vi "Agilent 6000 Series Edge Triggered Acquisition.vi"() -> ()   [LabVIEW 2017]
doc: "This example shows how to configure the oscilloscope to perform an edge-triggered waveform acquisition."
uses:
  <instrlib>/Agilent 6000 Series/Public/Configure/Configure Edge Trigger Source.vi
  <instrlib>/Agilent 6000 Series/Public/Data/Read Single Waveform.vi
  <instrlib>/Agilent 6000 Series/Agilent 6000 Series.lvlib
panel:
  in  "Channel (0: Channel 1)":u16(ring) items=["Channel 1", "Channel 2", "Channel 3", "Channel 4"]
  in  "Vertical Coupling (1: DC)":u16(ring)=1 items=["AC", "DC"]
  in  "Probe Attenuation (10.0)":dbl=10.0
  in  "Vertical Range (10.0 V)":dbl=10.0
  in  "Trigger Level (0.5 V)":dbl=0.5
  in  "Timebase (0.0005 s)":dbl=0.0005
  out "Waveform Data":waveform(dbl)(graph)
  in  "VISA resource name":refnum<visa-resource-name>
  # "(c) 2009-2015 National Instruments.  ALL RIGHTS RESERVED."
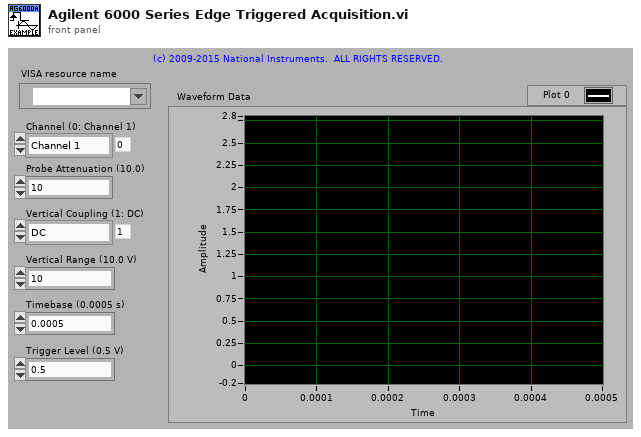
[diagram p1: front panel]
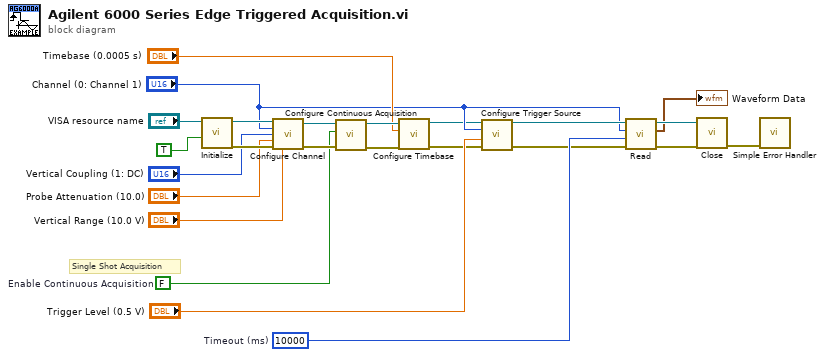
[diagram p0: block diagram]
diagram:
  w14 = u32 10000  # Timeout (ms)
  w9 = FALSE  # Enable Continuous Acquisition
  # "Single Shot Acquisition"
  n1 = call <instrlib>:"Initialize.vi"("Reset? (T: Yes)"=TRUE, "VISA resource name"="VISA resource name") -> ("error out"=w21:errorcluster, "VISA resource name out"=w22:refnum<visa-resource-name>)  [unwired: 8 in]
  n2 = call <instrlib>:"Configure Channel.vi"("VISA resource name"=w22, "Channel (0: Channel 1)"="Channel (0: Channel 1)", "Vertical Coupling (0: AC)"="Vertical Coupling (1: DC)", "Probe Attenuation (10.0)"="Probe Attenuation (10.0)", "error in (no error)"=w21, "Vertical Range (10.0 V)"="Vertical Range (10.0 V)") -> ("VISA resource name out"=w10:refnum<visa-resource-name>, "error out"=w13:errorcluster)  [unwired: 8 in]
  n3 = call <instrlib>:"Configure Continuous Acquisition.vi"("error in (no error)"=w13, "Continuous Acquisition Mode (T: Enable)"=w9, "VISA resource name"=w10) -> ("error out"=w12:errorcluster, "VISA resource name out"=w11:refnum<visa-resource-name>)  [unwired: 7 in]
  n4 = call <instrlib>:"Configure Timebase.vi"("error in (no error)"=w12, "Timebase (20.0E-9)"="Timebase (0.0005 s)", "VISA resource name"=w11) -> ("error out"=w1:errorcluster, "VISA resource name out"=w2:refnum<visa-resource-name>)  [unwired: 7 in]
  n5 = call-poly <instrlib>:"Configure Trigger Source.vi"("VISA resource name"=w2, "Trigger Source (0: Channel 1)"="Channel (0: Channel 1)", "Trigger Level (0.0 V)"="Trigger Level (0.5 V)", "error in (no error)"=w1) -> ("VISA resource name out"=w5:refnum<visa-resource-name>, "error out"=w6:errorcluster)  [unwired: 10 in]
  n6 = call-poly <instrlib>:"Read.vi"("error in (no error)"=w6, "Timeout (10000 ms)"=w14, "Source (0: Channel 1)"="Channel (0: Channel 1)", "VISA resource name"=w5) -> ("error out"=w19:errorcluster, "Waveform Data"=→"Waveform Data":waveform(dbl), "VISA resource name out"=w20:refnum<visa-resource-name>)  [unwired: 5 in]
  n7 = call <instrlib>:"Close.vi"("error in (no error)"=w19, "VISA resource name"=w20) -> ("error out"=w24:errorcluster)  [unwired: 9 in]
  n8 = call <vilib>:"Simple Error Handler.vi"("error in (no error)"=w24) -> ()  [unwired: 4 in, 5 out]
